vi "test_fit_SOS.vi"() -> ()   [LabVIEW 2017]
uses:
  controls/SOS_frf_data.ctl
  subVIs/auto-sys-id/fit_sos_results.ctl
  <vilib>/addons/_JKI.lib/Serialization/JSON/JKI JSON Serialization.lvlib
panel:
  out "error out 2":errorcluster
  out "fit_sos_result":T1
  out "theta 2":dbl[](array[numeric])
  out "element 2":dbl
  out "element":dbl
  out "results":dbl[](array[numeric])
  out "return type":i32
  out "theta":dbl[](array[numeric])
  out "error out":errorcluster
  out "frf_data":T2
  in  "error in (no error)":errorcluster
  in  "system data path":path=path "C:/Users/arnold/Documents/afm-cs/c-src/frf_test_data.json"
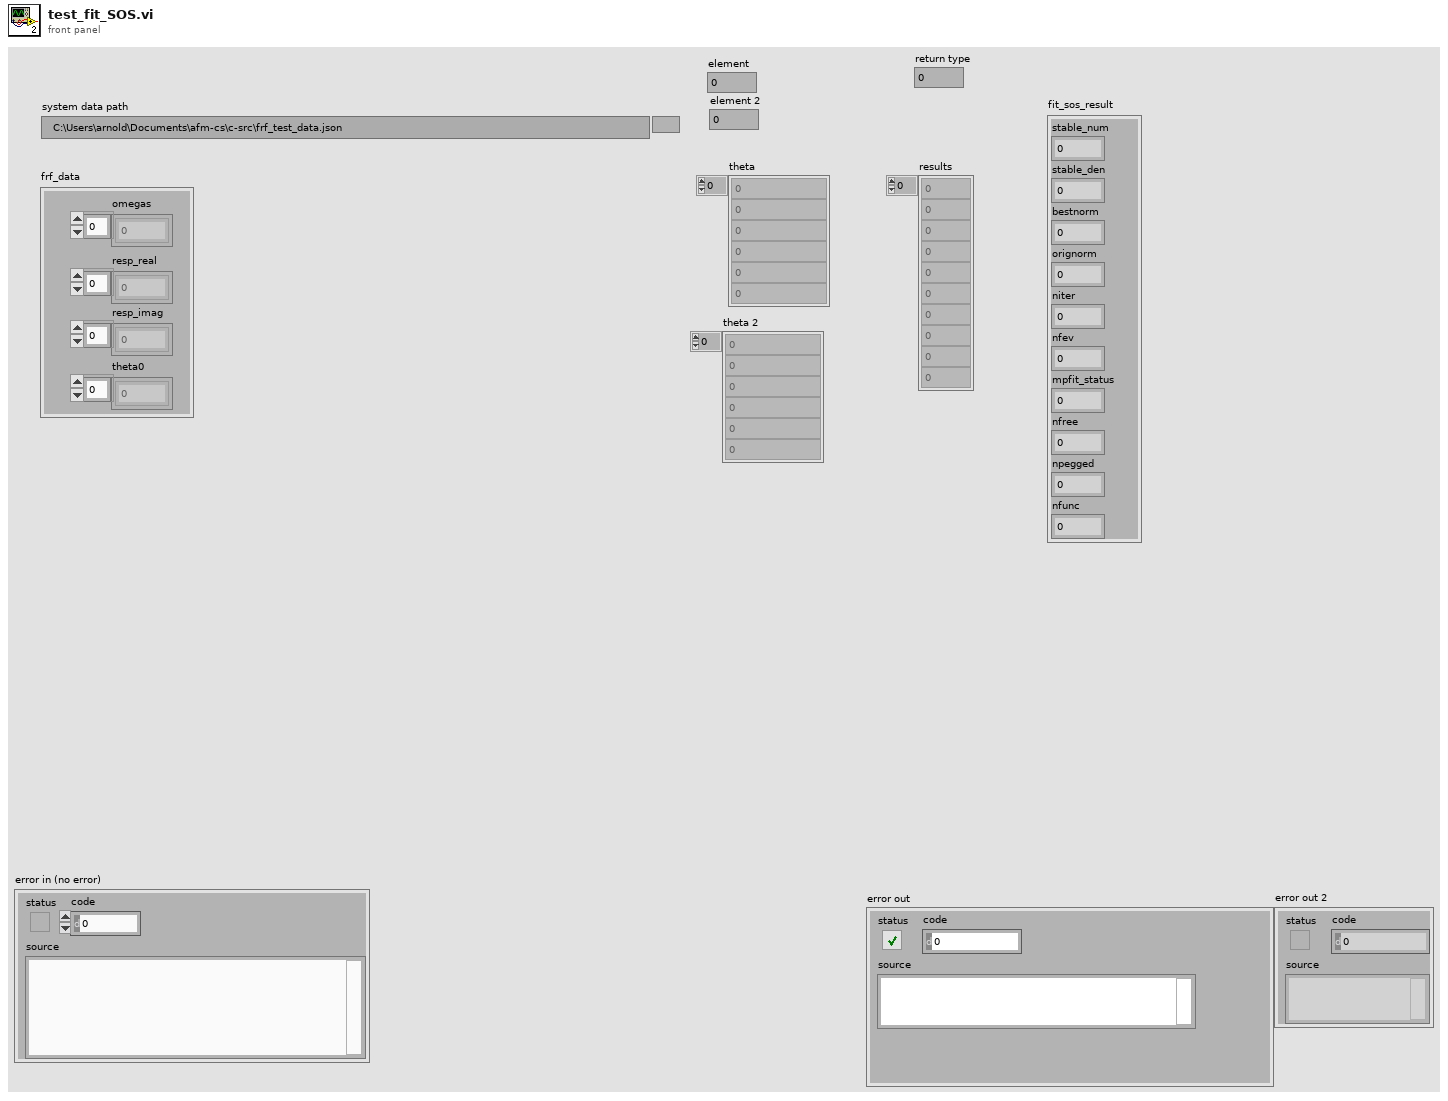
[diagram p1: front panel]
types:
  T1 = typedef "fit_sos_results.ctl" = cluster{"stable_num":i32, "stable_den":i32, "bestnorm":dbl, "orignorm":dbl, "niter":i32, "nfev":i32, "mpfit_status":i32, "nfree":i32, "npegged":i32, "nfunc":i32}
  T2 = typedef "SOS_frf_data.ctl" = cluster{"omegas":dbl[], "resp_real":dbl[], "resp_imag":dbl[], "theta0":dbl[]}
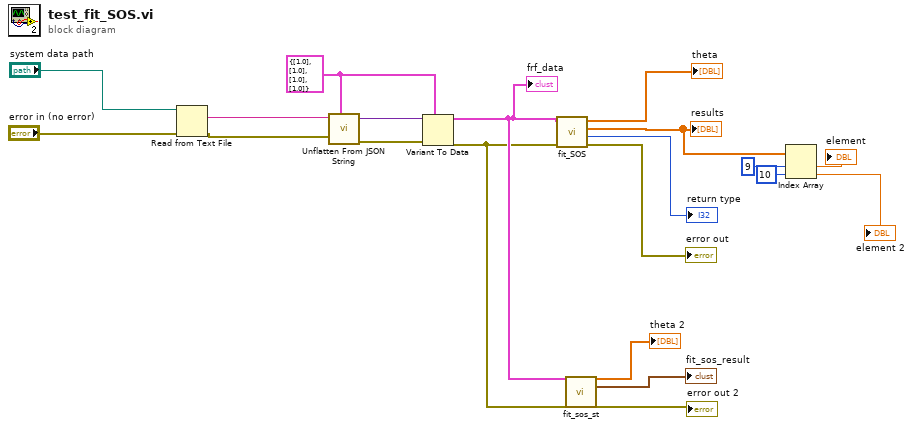
[diagram p0: block diagram]
diagram:
  w14 = T2 {"omegas"=[1.0], "resp_real"=[1.0], "resp_imag"=[1.0], "theta0"=[1.0]} ("frf_data")
  n1 = Read from Text File(file (use dialog)="system data path", error in="error in (no error)") -> (text=w18:string, error out=w17:errorcluster)  [unwired: 2 in, 2 out]
  n2 = call <vilib>:"Unflatten From JSON String.vi"("Type and Defaults"=w14, "error in (no error)"=w17, "JSON String"=w18) -> ("error out"=w19:errorcluster, "Variant"=w20:variant)  [unwired: 7 in]
  n3 = Variant To Data(error in=w19, type=w14, Variant=w20) -> (data=w5:T2, error out=w4:errorcluster)
  "frf_data" <- w5
  n4 = call "fit_SOS.vi"("error"=w4, "frf_data"=w5) -> ("error out"=→"error out":errorcluster, "return type"=→"return type":i32, "results"=w10:dbl[], "theta"=→"theta":dbl[])  [unwired: 6 in]
  "results" <- w10
  n5 = call "fit_sos_st.vi"("frf_data"=w5, "error in (no error)"=w4) -> ("theta"=→"theta 2":dbl[], "fit_sos_result"=→"fit_sos_result":T1, "error out"=→"error out 2":errorcluster)  [unwired: 23 in]
  n6 = Index Array(array=w10, index #1=9 ("index"), index #2=10 ("index")) -> (element #1=→"element":dbl, element #2=→"element 2":dbl)
